vi "Display Item Image.vi"(8 "error in (no error)":errorcluster, 10 "Color Image":T1, 11 "2D Picture Ref":refnum<vi>) -> (0 "error out":errorcluster)   [LabVIEW 2020, in "VI Properties Editor.lvlib"]
doc: "Displays <B>Color Image</B> to the picture control associated with <B>2D Picture Ref</B>, also showing scrollbars if needed and setting the origin to (0, 0)."
uses:
  VI Properties Editor.lvlib
  <vilib>/picture/picture.llb/imagedata.ctl
  <vilib>/Utility/miscctls.llb/LVPointTypeDef.ctl
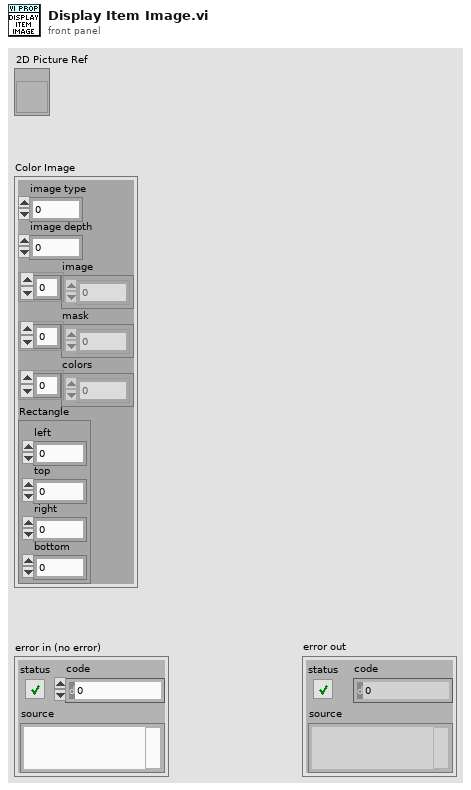
[diagram p1: front panel]
types:
  T1 = typedef "imagedata.ctl" = cluster{"image type":i32, "image depth":i32, "image":u8[], "mask":u8[], "colors":u32[], "Rectangle":cluster{"left":i16, "top":i16, "right":i16, "bottom":i16}}
  T2 = typedef "LVPointTypeDef.ctl" = cluster{"Horizontal":i16, "Vertical":i16}
  T3 = typedef "LVBoundsTypeDef.ctl" = cluster{"Width":u32, "Height":u32}
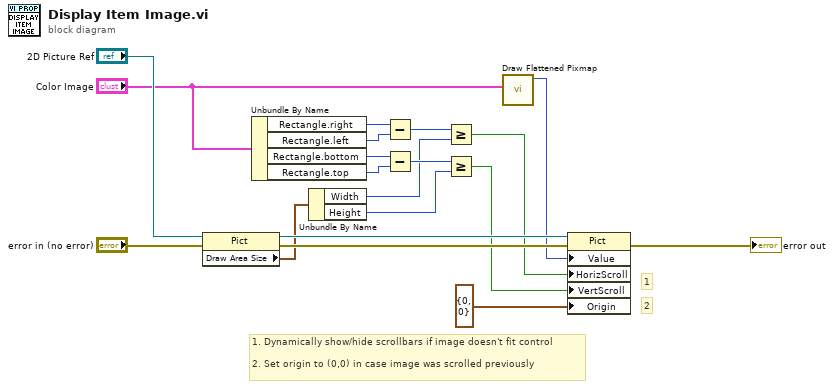
[diagram p0: block diagram]
diagram:
  # "1. Dynamically show/hide scrollbars if image doesn't fit control\n\n2. Set origin to (0,0) in case image was scrolled previously"
  # "2"
  # "1"
  n1 = property class="Pict"(reference="2D Picture Ref", error in="error in (no error)") -> (reference out=w18:refnum<vi>, error out=w17:errorcluster, "Draw Area Size"=w8:T3)
  n2 = Unbundle By Name("Color Image") -> ("Rectangle.right"=w13:i16, "Rectangle.left"=w12:i16, "Rectangle.bottom"=w11:i16, "Rectangle.top"=w10:i16)
  n3 = Unbundle By Name(w8) -> ("Width"=w5:u32, "Height"=w4:u32)
  n4 = Subtract(x=w13, y=w12) -> (x-y=w7:i16)
  n5 = Subtract(x=w11, y=w10) -> (x-y=w6:i16)
  n6 = Greater Or Equal?(x=w7, y=w5) -> (x >= y?=w3:bool)
  n7 = Greater Or Equal?(x=w6, y=w4) -> (x >= y?=w2:bool)
  n8 = call <vilib>:"Draw Flattened Pixmap.vi"("image data"="Color Image") -> ("new picture"=w14:picture)  [unwired: 8 in]
  n9 = property class="Pict"(reference=w18, error in=w17, "Value"=w14, "HorizScroll"=w3, "VertScroll"=w2, "Origin"=T2 {"Horizontal"=0, "Vertical"=0}) -> (error out=→"error out":errorcluster)  [unwired: 1 out]
